vi "Round Ceiling to Places.vi"(9 "Places In":i32, 11 "Float In":sgl) -> (3 "Float Out":sgl format="%.4f")   [LabVIEW 2024]
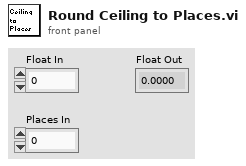
[diagram p1: front panel]
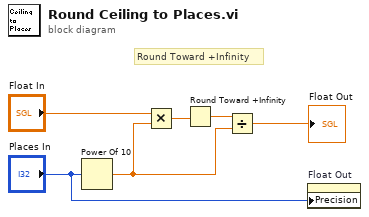
[diagram p0: block diagram]
diagram:
  # "Round Toward +Infinity"
  n1 = Power Of 10(x="Places In") -> (10^x=w3:dbl)
  n2 = Multiply(x="Float In", y=w3) -> (x*y=w5:dbl)
  n3 = Round Toward +Infinity(x=w5) -> (ceil(x): smallest int >= x=w4:dbl)
  n4 = Divide(x=w4, y=w3) -> (x/y=→"Float Out":dbl)
  n5 = property on="Float Out" class="DigNum (strict)"("Precision"="Places In") -> ()  [unwired: 2 in, 2 out]
